vi "Entity Identifier.vi"(11 "User in":refnum<class "User.lvclass">) -> (2 "Identifier Column":refnum<class "String.lvclass">)   [LabVIEW 2020, in "HTTP-Conditum.lvlib" / "User.lvclass"]
doc: "This VI is called to determine the column and value that a user entity uses to identify users. This will typically be whatever value is used for logging in such as a username or email address.\n\nIf the user entity already has an indentification value set it should be populated in the indentifier column that is returned."
uses:
  User.lvclass
  <vilib>/IlluminatedG/IG Conditum/Conditum/Columns/String/String.lvclass
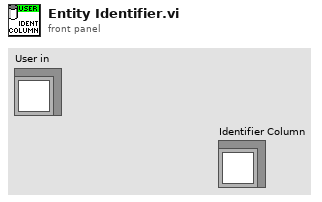
[diagram p1: front panel]
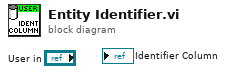
[diagram p0: block diagram]
diagram:
